vi "EvaluateSuit.vi"(4 "Count":u16[](array[numeric])) -> (0 "Pair":u16, 1 "Taatsu":u16, 2 "Meld":u16)   [LabVIEW 2025]
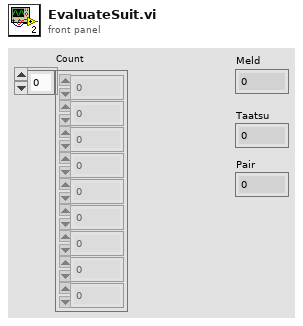
[diagram p1: front panel]
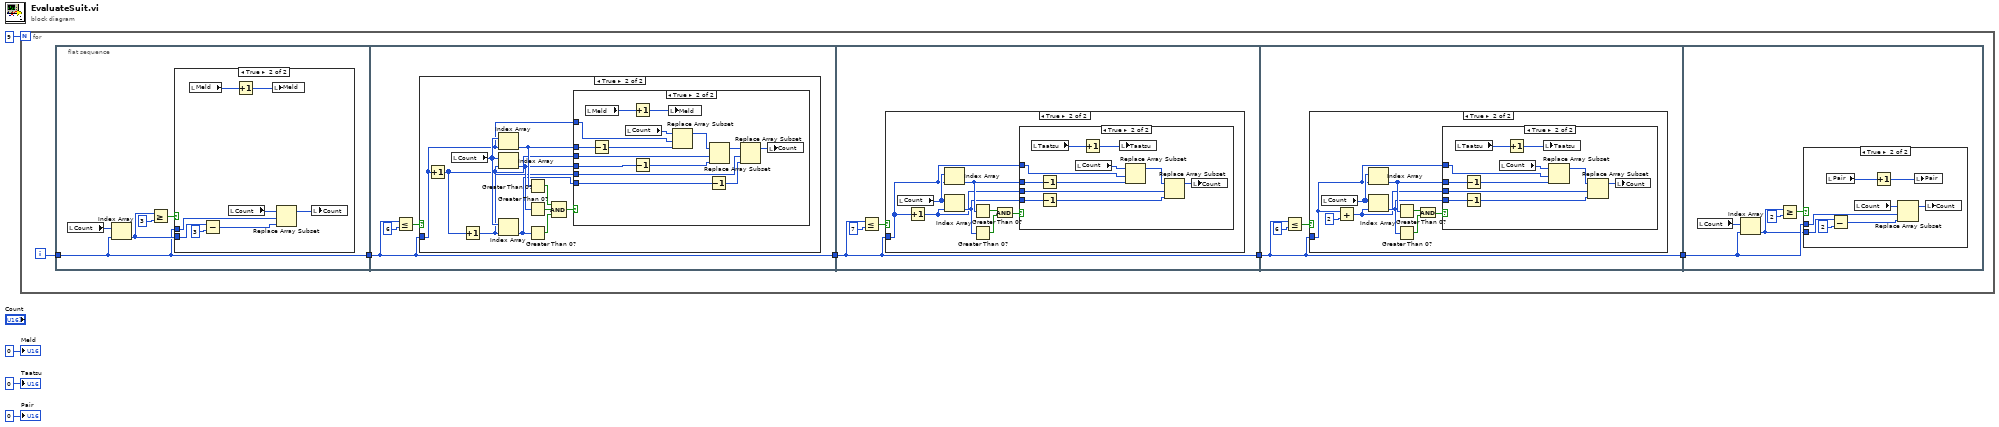
[diagram p0: block diagram]
diagram:
  n1 = for {
    N: 9 -> [_]
    i -> [w9]
    n2 = flat-sequence {
      tunnel: w9 -> [w10]
      tunnel: [w10] -> w8
      tunnel: w8 -> [w23]
      tunnel: [w23] -> w7
      tunnel: w7 -> [w52]
      tunnel: [w52] -> w6
      tunnel: w6 -> [w74]
      tunnel: [w74] -> w5
      tunnel: w5 -> [w98]
      frame #0 {
        n3 = local read "Count"() -> (w12:u16[])
        n4 = Index Array(array=w12, index=w10) -> (element=w14:u16)
        n5 = Greater Or Equal?(x=w14, y=3) -> (x >= y?=w13:bool)
        n6 = case shown="True" w13 {
          tunnel: w10 -> [_ w20]
          tunnel: w14 -> [_ w19]
          frame False {
          }
          frame True {
            n7 = local read "Meld"() -> (w15:u16)
            n8 = Subtract(x=w19, y=3) -> (x-y=w21:i32)
            n9 = local read "Count"() -> (w22:u16[])
            n10 = Increment(x=w15) -> (x+1=w16:u16)
            n11 = local write "Meld"(w16) -> ()
            n12 = Replace Array Subset(array=w22, new element=w21, index=w20) -> (w17:u16[])
            n13 = local write "Count"(w17) -> ()
          }
        }
      }
      frame #1 {
        n14 = Less Or Equal?(x=w23, y=6) -> (x <= y?=w25:bool)
        n15 = case shown="True" w25 {
          tunnel: w23 -> [_ w30]
          frame False {
          }
          frame True {
            n16 = Increment(x=w30) -> (x+1=w27:i32)
            n17 = local read "Count"() -> (w36:u16[])
            n18 = Increment(x=w27) -> (x+1=w26:i32)
            n19 = Index Array(array=w36, index=w30) -> (element=w31:u16)
            n20 = Index Array(array=w36, index=w27) -> (element=w29:u16)
            n21 = Index Array(array=w36, index=w26) -> (element=w28:u16)
            n22 = Greater Than 0?(x=w31) -> (x > 0?=w35:bool)
            n23 = Greater Than 0?(x=w29) -> (x > 0?=w34:bool)
            n24 = Greater Than 0?(x=w28) -> (x > 0?=w33:bool)
            n25 = Compound Arithmetic op=AND(w35, w34, w33) -> (w32:bool)
            n26 = case shown="True" w32 {
              tunnel: w30 -> [_ w48]
              tunnel: w31 -> [_ w46]
              tunnel: w27 -> [_ w44]
              tunnel: w26 -> [_ w41]
              tunnel: w29 -> [_ w39]
              tunnel: w28 -> [_ w37]
              frame False {
              }
              frame True {
                n27 = local read "Meld"() -> (w51:u16)
                n28 = Decrement(x=w46) -> (x-1=w47:u16)
                n29 = local read "Count"() -> (w49:u16[])
                n30 = Increment(x=w51) -> (x+1=w50:u16)
                n31 = Decrement(x=w39) -> (x-1=w40:u16)
                n32 = local write "Meld"(w50) -> ()
                n33 = Replace Array Subset(array=w49, new element=w47, index=w48) -> (w45:u16[])
                n34 = Decrement(x=w37) -> (x-1=w38:u16)
                n35 = Replace Array Subset(array=w45, new element=w40, index=w44) -> (w43:u16[])
                n36 = Replace Array Subset(array=w43, new element=w38, index=w41) -> (w42:u16[])
                n37 = local write "Count"(w42) -> ()
              }
            }
          }
        }
      }
      frame #2 {
        n38 = Less Or Equal?(x=w52, y=7) -> (x <= y?=w53:bool)
        n39 = case shown="True" w53 {
          tunnel: w52 -> [_ w57]
          frame False {
          }
          frame True {
            n40 = local read "Count"() -> (w62:u16[])
            n41 = Increment(x=w57) -> (x+1=w55:i32)
            n42 = Index Array(array=w62, index=w57) -> (element=w58:u16)
            n43 = Index Array(array=w62, index=w55) -> (element=w56:u16)
            n44 = Greater Than 0?(x=w58) -> (x > 0?=w61:bool)
            n45 = Greater Than 0?(x=w56) -> (x > 0?=w60:bool)
            n46 = And(x=w61, y=w60) -> (x .and. y?=w59:bool)
            n47 = case shown="True" w59 {
              tunnel: w57 -> [_ w70]
              tunnel: w58 -> [_ w68]
              tunnel: w56 -> [_ w65]
              tunnel: w55 -> [_ w63]
              frame False {
              }
              frame True {
                n48 = local read "Taatsu"() -> (w73:u16)
                n49 = Decrement(x=w68) -> (x-1=w69:u16)
                n50 = Decrement(x=w65) -> (x-1=w66:u16)
                n51 = local read "Count"() -> (w71:u16[])
                n52 = Increment(x=w73) -> (x+1=w72:u16)
                n53 = local write "Taatsu"(w72) -> ()
                n54 = Replace Array Subset(array=w71, new element=w69, index=w70) -> (w67:u16[])
                n55 = Replace Array Subset(array=w67, new element=w66, index=w63) -> (w64:u16[])
                n56 = local write "Count"(w64) -> ()
              }
            }
          }
        }
      }
      frame #3 {
        n57 = Less Or Equal?(x=w74, y=6) -> (x <= y?=w76:bool)
        n58 = case shown="True" w76 {
          tunnel: w74 -> [_ w78]
          frame False {
          }
          frame True {
            n59 = local read "Count"() -> (w85:u16[])
            n60 = Add(x=w78, y=2) -> (x+y=w79:i32)
            n61 = Index Array(array=w85, index=w78) -> (element=w81:u16)
            n62 = Index Array(array=w85, index=w79) -> (element=w80:u16)
            n63 = Greater Than 0?(x=w81) -> (x > 0?=w84:bool)
            n64 = Greater Than 0?(x=w80) -> (x > 0?=w83:bool)
            n65 = And(x=w84, y=w83) -> (x .and. y?=w82:bool)
            n66 = case shown="True" w82 {
              tunnel: w78 -> [_ w93]
              tunnel: w81 -> [_ w91]
              tunnel: w80 -> [_ w88]
              tunnel: w79 -> [_ w86]
              frame False {
              }
              frame True {
                n67 = local read "Taatsu"() -> (w96:u16)
                n68 = Decrement(x=w91) -> (x-1=w92:u16)
                n69 = Decrement(x=w88) -> (x-1=w89:u16)
                n70 = local read "Count"() -> (w94:u16[])
                n71 = Increment(x=w96) -> (x+1=w95:u16)
                n72 = local write "Taatsu"(w95) -> ()
                n73 = Replace Array Subset(array=w94, new element=w92, index=w93) -> (w90:u16[])
                n74 = Replace Array Subset(array=w90, new element=w89, index=w86) -> (w87:u16[])
                n75 = local write "Count"(w87) -> ()
              }
            }
          }
        }
      }
      frame #4 {
        n76 = local read "Count"() -> (w101:u16[])
        n77 = Index Array(array=w101, index=w98) -> (element=w97:u16)
        n78 = Greater Or Equal?(x=w97, y=u16 2) -> (x >= y?=w99:bool)
        n79 = case shown="True" w99 {
          tunnel: w98 -> [_ w108]
          tunnel: w97 -> [_ w105]
          frame False {
          }
          frame True {
            n80 = local read "Pair"() -> (w102:u16)
            n81 = Subtract(x=w105, y=u16 2) -> (x-y=w106:u16)
            n82 = local read "Count"() -> (w109:u16[])
            n83 = Increment(x=w102) -> (x+1=w103:u16)
            n84 = Replace Array Subset(array=w109, new element=w106, index=w108) -> (w107:u16[])
            n85 = local write "Pair"(w103) -> ()
            n86 = local write "Count"(w107) -> ()
          }
        }
      }
    }
  }
  "Meld" <- u16 0 ("Meld")
  "Taatsu" <- u16 0 ("Taatsu")
  "Pair" <- u16 0 ("Pair")
